vi "HW GV.vi"() -> ()   [LabVIEW 2019, in "HW Control.lvlib"]
uses:
  HW Control.lvlib
panel:
  in  "HW Status":string
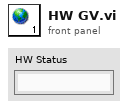
[diagram p1: front panel]
diagram:
